vi "题目6.vi"() -> ()   [LabVIEW 2017]
panel:
  out "日期/时间字符串":string
  in  "时间格式字符串(%c)":string
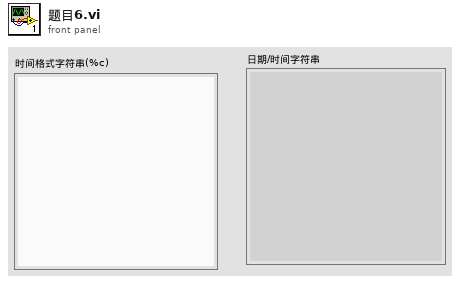
[diagram p1: front panel]
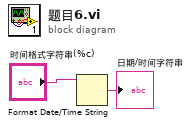
[diagram p0: block diagram]
diagram:
  n1 = Format Date/Time String(time format string (%c)="时间格式字符串(%c)") -> (date/time string=→"日期/时间字符串":string)  [unwired: 2 in]
